vi "Variant Array Elements.vi"(8 "error in (no error)":errorcluster, 11 "N Dim Array":variant) -> (0 "error out":errorcluster, 1 "Element Type":variant, 2 "Sizes":i32[](array[numeric]), 3 "Elements":variant[](array[variant]))   [LabVIEW 2019, in "labview_json.lvlib"]
uses:
  labview_json.lvlib
  <vilib>/Utility/error.llb/Error Cluster From Error Code.vi
  <vilib>/ErrorRing/Error Ring.xnode
  <vilib>/Utility/Data Type/NI_Data Type.lvlib
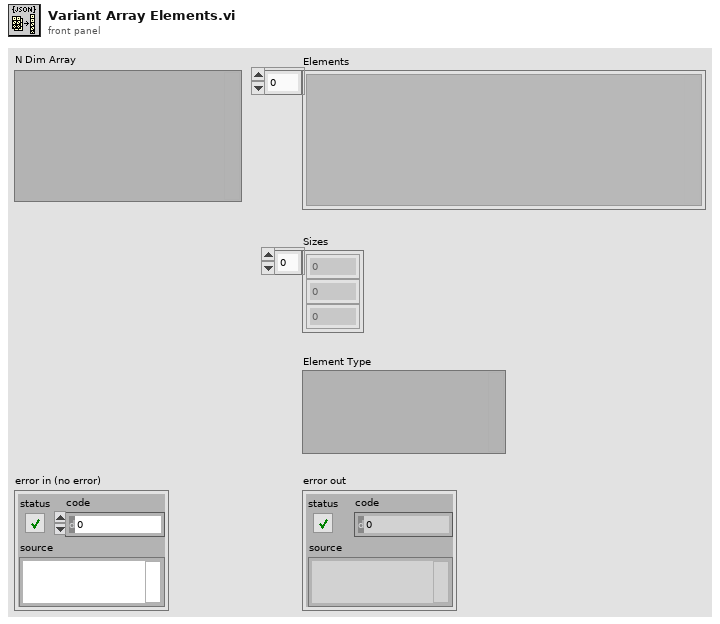
[diagram p1: front panel]
types:
  T1 = typedef "NI_Data Type.lvlib/Data Type.ctl" = enum8{"Invalid Type", "Void", "I8", "I16", "I32", "I64", "U8", "U16", "U32", "U64", "Single Float", "Double Float", "Extended Float", "Single Complex", "Double Complex", "Extended Complex", "Enum U8", "Enum U16", "Enum U32", "Enum U64", "Single Float With Unit", "Double Float With Unit", "Extended Float With Unit", "Single Complex with Unit", "Double Complex with Unit", "Extended Complex with Unit", "Boolean", "String", "Path", "Picture", "Tag", "Array", "Cluster", "Variant", "LV Variant", "Waveform", "Timestamp", "Digital Waveform", "Digital Data", "ExpressData", "Refnum", "External Data", "VI", "Poly VI", "LabVIEW Class Instance", "Fixed Point", "Set Collection", "Map Collection"}
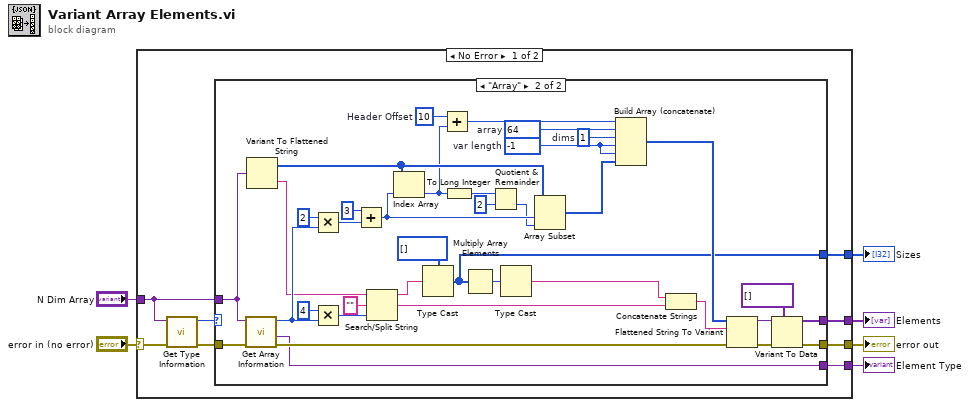
[diagram p0: block diagram]
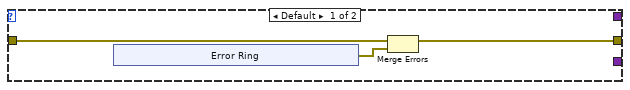
[diagram p2: hidden frame]
diagram:
  n1 = case shown="No Error" "error in (no error)" {
    selector: "error in (no error)" -> [w14 w59]
    tunnel: [w12 w59] -> w5
    tunnel: "N Dim Array" -> [w11 _]
    tunnel: [w9 _] -> w3
    tunnel: [w8 _] -> w2
    tunnel: [w7 _] -> w1
    frame No Error {
      n2 = call <vilib>:"Get Type Information.vi"("error in (no error)"=w14, "variant"=w11) -> ("error out"=w13:errorcluster, "type"=w10:T1)  [unwired: 5 in, 3 out]
      n3 = case shown="\"Array\"" w10 {
        tunnel: w13 -> [w17 w58]
        tunnel: [w16 w25] -> w12
        tunnel: w11 -> [_ w57]
        tunnel: [_ w23] -> w9
        tunnel: [_ w27] -> w8
        tunnel: [_ w26] -> w7
        frame Default {
          n4 = xnode "Error Ring"() -> ("error out"=w15:errorcluster)
          n5 = Merge Errors(w17, w15) -> (w16:errorcluster)
        }
        frame "Array" {
          w39 = i16 -1  # var length
          w40 = i16 1  # dims
          w46 = i16 10  # Header Offset
          w53 = i16 64  # array
          n6 = call <vilib>:"Get Array Information.vi"("error in (no error)"=w58, "variant"=w57) -> ("error out"=w37:errorcluster, "array element data type"=w26:variant, "number of dimensions"=w42:i32)  [unwired: 6 in, 1 out]
          n7 = Variant To Flattened String(Variant=w57) -> (data string=w41:string, 1:w52:i16[])
          n8 = Multiply(x=2, y=w42) -> (x*y=w55:i32)
          n9 = Multiply(x=4, y=w42) -> (x*y=w30:i32)
          n10 = Add(x=3, y=w55) -> (x+y=w51:i32)
          n11 = Search/Split String(string=w41, search string/char (-)="", offset (0)=w30) -> (substring before match=w29:string, match + rest of string=w33:string)  [unwired: 1 out]
          n12 = Index Array(array=w52, index=w51) -> (element=w47:i16)
          n13 = Type Cast(type=i32[] [], x=w29) -> (*(type *) &x=w27:i32[])
          n14 = Add(x=w46, y=w47) -> (x+y=w45:i16)
          n15 = To Long Integer(number=w47) -> (32bit integer=w49:i32)
          n16 = Multiply Array Elements(1:w27) -> (0:w44:i32)
          n17 = Quotient & Remainder(x=w49, y=2) -> (floor(x/y)=w48:i32)  [unwired: 1 out]
          n18 = Type Cast(x=w44) -> (*(type *) &x=w34:string)  [unwired: 1 in]
          n19 = Array Subset(array=w52, index=w51, length=w48) -> (w38:i16[])
          n20 = Build Array (concatenate)(w45, w53, w40, w39, w39, w38) -> (w35:i16[])
          n21 = Concatenate Strings(w34, w33) -> (w32:string)
          n22 = Flattened String To Variant(4:w37, 6:w32, 7:w35) -> (0:w36:errorcluster, 3:w24:variant)
          n23 = Variant To Data(error in=w36, type=variant[] [], Variant=w24) -> (data=w23:variant[], error out=w25:errorcluster)
        }
      }
    }
    frame Error {
    }
  }
  "error out" <- w5
  "Elements" <- w3
  "Sizes" <- w2
  "Element Type" <- w1
